vi "Get Mean Free Path.vi"(1 "P":dbl, 2 "T":dbl) -> (0 "l (mm)":dbl)   [LabVIEW 2014, in "Atmospheric Library.lvlib"]
doc: "This function returns the mean free path of air as a function of temperature and pressure."
uses:
  Atmospheric Library.lvlib
  Atmospheric Constants.vi
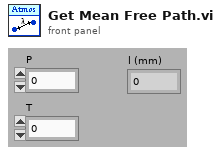
[diagram p1: front panel]
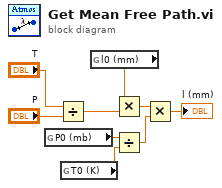
[diagram p0: block diagram]
diagram:
  n1 = global read "Atmospheric Constants.vi" "P0 (mb)"() -> (w9:sgl)
  n2 = Divide(x="T", y="P") -> (x/y=w5:dbl)
  n3 = global read "Atmospheric Constants.vi" "T0 (K)"() -> (w8:sgl)
  n4 = global read "Atmospheric Constants.vi" "l0 (mm)"() -> (w4:dbl)
  n5 = Multiply(x=w4, y=w5) -> (x*y=w3:dbl)
  n6 = Divide(x=w9, y=w8) -> (x/y=w2:sgl)
  n7 = Multiply(x=w3, y=w2) -> (x*y=→"l (mm)":dbl)
